vi "actuate_PairedPulseExp_v0.04.vi"(0 "Phase Cluster":T4, 1 "valve Time Cluster":T3, 2 "Didn't Lift?":bool, 3 "data in":T5={"daq_ao 1"="Dev1/ao0", "daq_ai 1"="Dev1/ai0", "experiment day folder"=path "D:/DATA/8-27-15 save func testing/test.lvm", "Multiclamp init error"=0, "Multiclamp Handle Out"=0, "sampling rate (Hz)"=10000, "trial name"=""}, 5 "PhaseLetter":string, 7 "controls array in":refnum<vi>[](array[refnum]), 9 "time to wait for solution change (min)":dbl=2.5 min=0.0 step=0.01, 11 "error in":errorcluster, 12 "common cluster":T7, 13 "individual controls in":T6) -> (4 "output cluster":T1, 6 "protocol waveform":waveform(dbl)[](graph), 8 "jumptestMonitor":waveform(dbl)[](graph) caption="protocol response", 10 "control array out":refnum<vi>[](array[refnum]), 14 "experiment VI ref":refnum<vi>, 15 "error out":errorcluster)   [LabVIEW 2019]
uses:
  pipette cleaning/pressure box/cleaning_soft/controls/actuator_type.ctl
  pipette cleaning/pressure box/cleaning_soft/controls/actuator_cluster.ctl
  machine_vision/coordinate model vis/transform_properties_actuators.ctl
  machine_vision/controls/transform_cluster_actuator.ctl
  controls/NH_method.ctl
  pipette cleaning/pressure box/cleaning_soft/controls/pressure_box_type.ctl
  pipette cleaning/pressure box/cleaning_soft/controls/pressure_box_control.ctl
  multipatch/controls/multipatch_common_controls_v4.ctl
  controls/memtest_def.ctl
  multipatch/controls/multipatch_individual_controls_v5.ctl
  Controls/Data.ctl
panel:
  in  "PairedPulseValuesCluster":T2
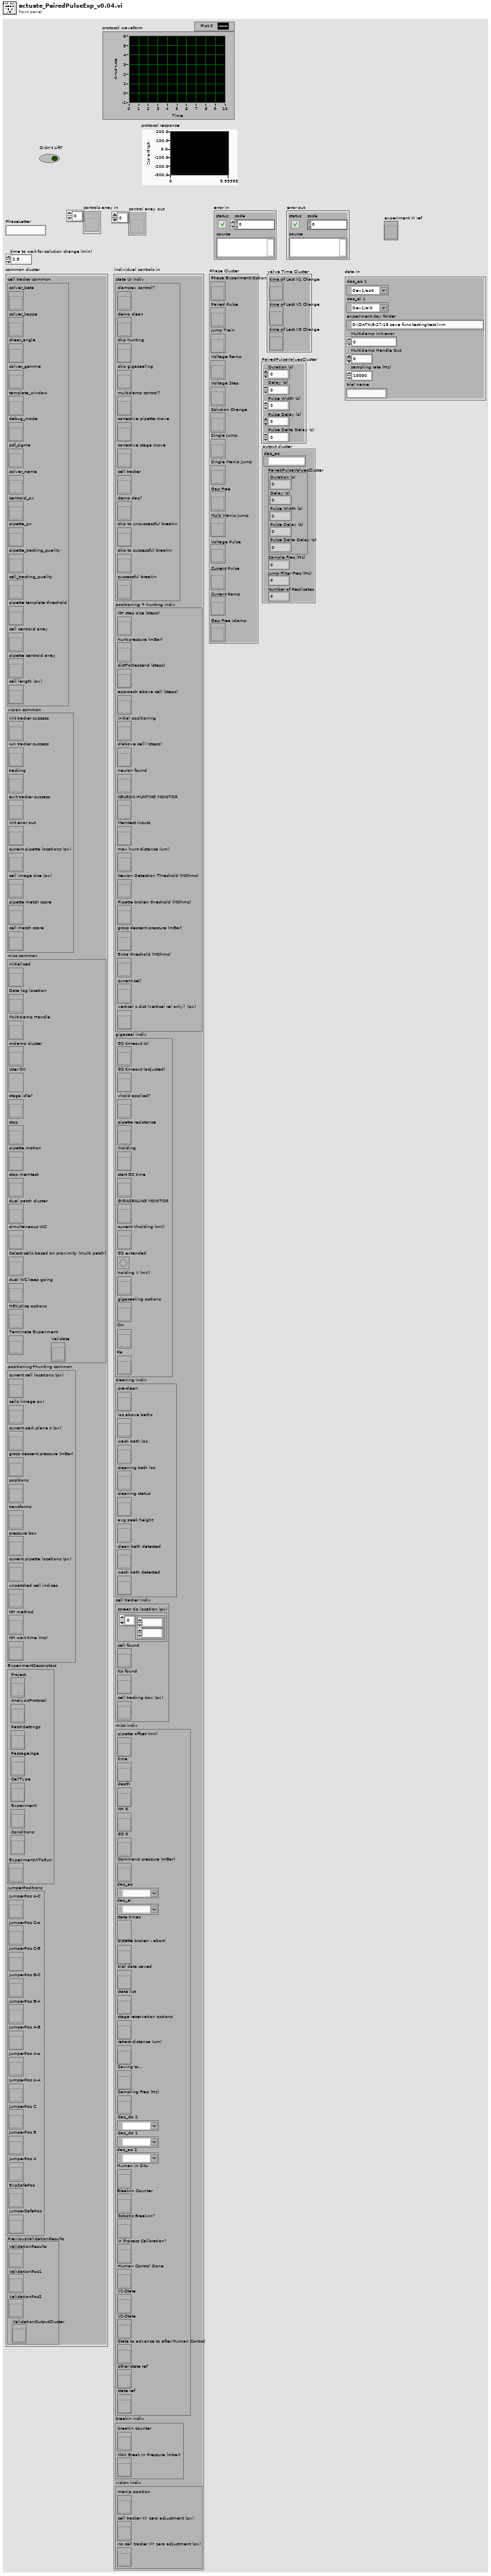
[diagram p1: front panel]
types:
  T1 = cluster{"daq_ao":tag, "PairedPulseValuesCluster":cluster{"Duration (s)":dbl, "Delay (s)":dbl, "Pulse Width (s)":dbl, "Pulse Delay (s)":dbl, "Pulse Delta Delay (s)":dbl}, "Sample Freq (Hz)":dbl, "Jump Filter Freq (Hz)":dbl, "Number of Replicates":i16}
  T2 = cluster{"Duration (s)":dbl, "Delay (s)":dbl, "Pulse Width (s)":dbl, "Pulse Delay (s)":dbl, "Pulse Delta Delay (s)":dbl}
  T3 = cluster{"time of Last V1 Change":refnum<vi>, "time of Last V2 Change":refnum<vi>, "time of Last V3 Change":refnum<vi>}
  T4 = cluster{"Phase Experiment Option":refnum<vi>, "Paired Pulse":refnum<vi>, "Jump Train":refnum<vi>, "Voltage Ramp":refnum<vi>, "Voltage Step":refnum<vi>, "Solution Change":refnum<vi>, "Single Jump":refnum<vi>, "Single Manip Jump":refnum<vi>, "Gap Free":refnum<vi>, "Multi Manip Jump":refnum<vi>, "Voltage Pulse":refnum<vi>, "Current Pulse":refnum<vi>, "Current Ramp":refnum<vi>, "Gap Free Iclamp":refnum<vi>}
  T5 = typedef "Data.ctl" = cluster{"daq_ao 1":tag, "daq_ai 1":tag, "experiment day folder":path, "Multiclamp init error":i32, "Multiclamp Handle Out":u32, "sampling rate (Hz)":i32, "trial name":string}
  T6 = typedef "multipatch_individual_controls_v5.ctl" = cluster{"state UI indiv":cluster{"clampex control?":refnum<vi>, "demo clean":refnum<vi>, "skip hunting":refnum<vi>, "skip gigasealing":refnum<vi>, "multiclamp control?":refnum<vi>, "corrective pipette move":refnum<vi>, "corrective stage move":refnum<vi>, "cell tracker":refnum<vi>, "demo daq?":refnum<vi>, "skip to unsuccessful breakin":refnum<vi>, "skip to successful breakin":refnum<vi>, "successful breakin":refnum<vi>}, "positioning + hunting indiv":cluster{"NH step size (steps)":refnum<vi>, "hunt pressure (mBar)":refnum<vi>, "distToDescend (steps)":refnum<vi>, "approach above cell (steps)":refnum<vi>, "initial positioning":refnum<vi>, "d(above cell) (steps)":refnum<vi>, "neuron found":refnum<vi>, "NEURON HUNTING MONITOR":refnum<vi>, "Memtest inputs":refnum<vi>, "max hunt distance (um)":refnum<vi>, "Neuron Detection Threshold (MOhms)":refnum<vi>, "Pipette broken threshold (MOhms)":refnum<vi>, "gross descent pressure (mBar)":refnum<vi>, "Extra threshold (MOhms)":refnum<vi>, "current cell":refnum<vi>, "vertical z dist (vertical rel only)  (px)":refnum<vi>}, "gigaseal indiv":cluster{"GS timeout (s)":refnum<vi>, "GS timeout (adjusted)":refnum<vi>, "vhold applied?":refnum<vi>, "pipette resistance":refnum<vi>, "Iholding":refnum<vi>, "start GS time":refnum<vi>, "GIGASEALING MONITOR":refnum<vi>, "current Vholding (mV)":refnum<vi>, "GS extended":refnum<vi>, "holding V (mV)":refnum<vi>, "gigasealing options":refnum<vi>, "Cm":refnum<vi>, "Ra ":refnum<vi>}, "cleaning indiv":cluster{"pre-clean":refnum<vi>, "loc above baths":refnum<vi>, "wash bath loc":refnum<vi>, "cleaning bath loc":refnum<vi>, "cleaning status":refnum<vi>, "avg peak height":refnum<vi>, "clean bath detected":refnum<vi>, "wash bath detected":refnum<vi>}, "cell tracker indiv":cluster{"screen tip location (px)":refnum<vi>, "cell found":refnum<vi>, "tip found":refnum<vi>, "cell tracking box (px)":refnum<vi>}, "misc indiv":cluster{"pipette offset (mV)":refnum<vi>, "time":refnum<vi>, "depth":refnum<vi>, "NH R":refnum<vi>, "GS R":refnum<vi>, "Command pressure (mBar)":refnum<vi>, "daq_ao":tag, "daq_ai":tag, "state times":refnum<vi>, "pipette broken - abort!":refnum<vi>, "trial data saved":refnum<vi>, "state list":refnum<vi>, "stage reservation options":refnum<vi>, "retract distance (um)":refnum<vi>, "Saving to...":refnum<vi>, "Sampling Freq (Hz)":refnum<vi>, "daq_do 2":tag, "daq_do 1":tag, "daq_ao 2":tag, "Human in Situ":refnum<vi>, "Break-In Counter":refnum<vi>, "Robotic Break-In?":refnum<vi>, "In Process Calibration?":refnum<vi>, "Human Control Done":refnum<vi>, "V1-State":refnum<vi>, "V2-State":refnum<vi>, "State to advance to after Human Control":refnum<vi>, "other state ref":refnum<vi>, "state ref":refnum<vi>}, "breakin indiv":cluster{"breakin counter":refnum<vi>, "MAX Break In Pressure (mbar)":refnum<vi>}, "vision indiv":cluster{"manip position":refnum<vi>, "cell tracker XY zero adjustment (px)":refnum<vi>, "no cell tracker XY zero adjustment (px)":refnum<vi>}}
  T7 = typedef "multipatch_common_controls_v4.ctl" = cluster{"cell tracker common":cluster{"solver_beta":refnum<vi>, "solver_kappa":refnum<vi>, "shear_angle":refnum<vi>, "solver_gamma":refnum<vi>, "template_window":refnum<vi>, "debug_mode":refnum<vi>, "psf_sigma":refnum<vi>, "solver_name":refnum<vi>, "centroid_px":refnum<vi>, "pipette_px":refnum<vi>, "pipette_tracking_quality":refnum<vi>, "cell_tracking_quality":refnum<vi>, "pipette template threshold":refnum<vi>, "cell centroid array":refnum<vi>, "pipette centroid array":refnum<vi>, "cell length (px)":refnum<vi>}, "vision common":cluster{"init tracker success":refnum<vi>, "run tracker success":refnum<vi>, "tracking":refnum<vi>, "exit tracker success":refnum<vi>, "init error out":refnum<vi>, "current pipette locations (px)":refnum<vi>, "cell image size (px)":refnum<vi>, "pipette match score":refnum<vi>, "cell match score":refnum<vi>}, "misc common":cluster{"initialized":refnum<vi>, "Data log location":refnum<vi>, "Multiclamp Handle":refnum<vi>, "mclamp cluster":refnum<vi>, "User OK":refnum<vi>, "stage idle?":refnum<vi>, "stop":refnum<vi>, "pipette motion":refnum<vi>, "stop memtest":refnum<vi>, "dual patch cluster":refnum<vi>, "simultaneous WC":refnum<vi>, "Select cells based on proximity (multi patch)":refnum<vi>, "dual WC keep going":refnum<vi>, "HEK/slice options":refnum<vi>, "Terminate Experiment":refnum<vi>, "Validate":refnum<vi>}, "positioning+hunting common":cluster{"current cell locations (px)":refnum<vi>, "cells (image px)":refnum<vi>, "current park plane z (px)":refnum<vi>, "gross descent pressure (mBar)":refnum<vi>, "positions":refnum<vi>, "transforms":refnum<vi>, "pressure box":refnum<vi>, "current pipette locations (px)":refnum<vi>, "unpatched cell indices":refnum<vi>, "NH method":refnum<vi>, "NH wait time (ms)":refnum<vi>}, "ExperimentDescriptors":cluster{"Project":refnum<vi>, "AnalysisProtocol":refnum<vi>, "PatchSettings":refnum<vi>, "Passage/Age":refnum<vi>, "CellType":refnum<vi>, "Experiment":refnum<vi>, "Conditions":refnum<vi>, "ExperimentVIToRun":refnum<vi>}, "JumperPositions":cluster{"JumperPos o-C":refnum<vi>, "JumperPos C-o":refnum<vi>, "JumperPos C-B":refnum<vi>, "JumperPos B-C":refnum<vi>, "JumperPos B-A":refnum<vi>, "JumperPos A-B":refnum<vi>, "JumperPos A-o":refnum<vi>, "JumperPos o-A":refnum<vi>, "JumperPos C":refnum<vi>, "JumperPos B":refnum<vi>, "JumperPos A":refnum<vi>, "ExpSafePos":refnum<vi>, "jumperSafePos":refnum<vi>}, "PreviousValidationResults":cluster{"ValidationResults":refnum<vi>, "ValidationPos1":refnum<vi>, "ValidationPos2":refnum<vi>, "ValidationOutputCluster":refnum<vi>}}
  T8 = cluster{"Which Position to use for Experiment":enum16{"Jumper Safe Position", "Experiment Safe Position", "Jumper Position A", "Jumper Position B", "Jumper Position C", "Jumper Position o-A", "Jumper Position A-o", "Jumper Position A-B", "Jumper Position B-A", "Jumper Position B-C", "Jumper Position C-B", "Jumper Position C-o", "Jumper Position o-C", "Don't Move"}, "Start Position (N)":string, "Jump Position (m)":string, "Duration (s)":dbl, "Delay (s)":dbl, "Pulse Width (s)":dbl, "Replicates":dbl, "Pulse Delay (s)":dbl, "Pulse Delta Delay (s)":dbl, "Vholding (mV)":dbl, "Valve 1 Position":i16, "Valve 2 Position":i16, "valve 1 used now?":bool, "valve 2 used now?":bool, "valve 3 used now? ":bool, "Valve 3 Position":i16, "protocol Preview":waveform(dbl)[]}
  T9 = enum16{"Jumper Safe Position", "Experiment Safe Position", "Jumper Position A", "Jumper Position B", "Jumper Position C", "Jumper Position o-A", "Jumper Position A-o", "Jumper Position A-B", "Jumper Position B-A", "Jumper Position B-C", "Jumper Position C-B", "Jumper Position C-o", "Jumper Position o-C", "Don't Move"}
  T10 = enum16{"manipulator 1", "manipulator 2", "manipulator 3", "manipulator 4"}
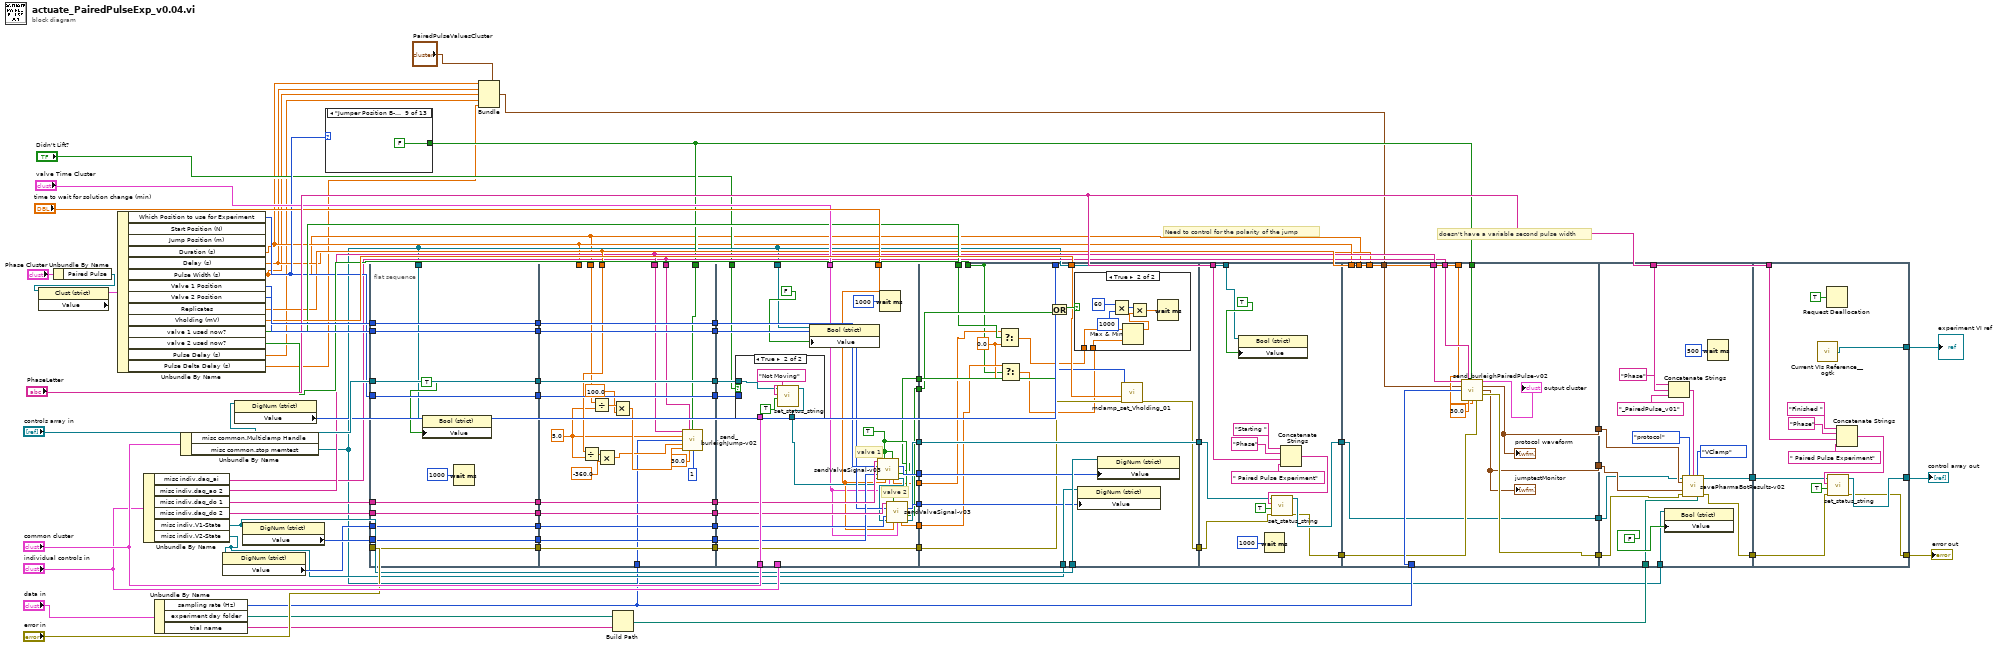
[diagram p0: block diagram]
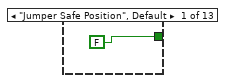
[diagram p2: hidden frame]
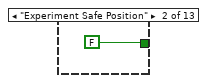
[diagram p3: hidden frame]
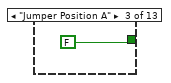
[diagram p4: hidden frame]
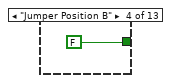
[diagram p5: hidden frame]
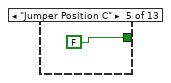
[diagram p6: hidden frame]
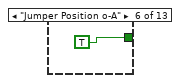
[diagram p7: hidden frame]
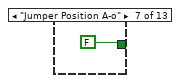
[diagram p8: hidden frame]
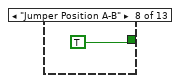
[diagram p9: hidden frame]
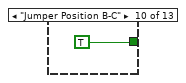
[diagram p10: hidden frame]
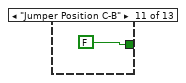
[diagram p11: hidden frame]
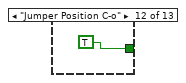
[diagram p12: hidden frame]
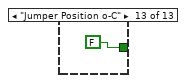
[diagram p13: hidden frame]
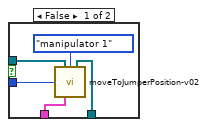
[diagram p14: hidden frame]
diagram:
  # "doesn't have a variable second pulse width"
  # "Need to control for the polarity of the jump"
  n1 = Unbundle By Name("Phase Cluster") -> ("Paired Pulse"=w59:refnum<vi>)
  n2 = property class="Clust (strict)"(reference=w59) -> ("Value"=w58:T8)  [unwired: 1 in, 2 out]
  n3 = Unbundle By Name(w58) -> ("Which Position to use for Experiment"=w34:T9, "Duration (s)"=w8:dbl, "Delay (s)"=w7:dbl, "Pulse Width (s)"=w6:dbl, "Valve 1 Position"=w57:i16, "Valve 2 Position"=w56:i16, "Replicates"=w24:dbl, "Vholding (mV)"=w43:dbl, "valve 1 used now?"=w36:bool, "valve 2 used now?"=w35:bool, "Pulse Delay (s)"=w5:dbl, "Pulse Delta Delay (s)"=w4:dbl)  [unwired: 2 out]
  n4 = Unbundle By Name("individual controls in") -> ("misc indiv.daq_ai"=w21:tag, "misc indiv.daq_ao 2"=w22:tag, "misc indiv.daq_do 1"=w79:tag, "misc indiv.daq_do 2"=w78:tag, "misc indiv.V1-State"=w70:refnum<vi>, "misc indiv.V2-State"=w69:refnum<vi>)
  n5 = Unbundle By Name("data in") -> ("sampling rate (Hz)"=w23:i32, "experiment day folder"=w63:path, "trial name"=w62:string)
  n6 = Unbundle By Name("common cluster") -> ("misc common.Multiclamp Handle"=w42:refnum<vi>, "misc common.stop memtest"=w10:refnum<vi>)
  n7 = property class="DigNum (strict)"(reference=w69) -> ("Value"=w71:u16)  [unwired: 1 in, 2 out]
  n8 = property class="DigNum (strict)"(reference=w42) -> ("Value"=w41:u32)  [unwired: 1 in, 2 out]
  n9 = property class="DigNum (strict)"(reference=w70) -> ("Value"=w72:u16)  [unwired: 1 in, 2 out]
  n10 = case shown="\"Jumper Position B-A\"" w34 {
    tunnel: [FALSE FALSE FALSE FALSE FALSE TRUE FALSE TRUE FALSE TRUE FALSE TRUE FALSE] -> w20
    frame "Jumper Safe Position", Default {
    }
    frame "Experiment Safe Position" {
    }
    frame "Jumper Position A" {
    }
    frame "Jumper Position B" {
    }
    frame "Jumper Position C" {
    }
    frame "Jumper Position o-A" {
    }
    frame "Jumper Position A-o" {
    }
    frame "Jumper Position A-B" {
    }
    frame "Jumper Position B-A" {
    }
    frame "Jumper Position B-C" {
    }
    frame "Jumper Position C-B" {
    }
    frame "Jumper Position C-o" {
    }
    frame "Jumper Position o-C" {
    }
  }
  n11 = flat-sequence {
    tunnel: "controls array in" -> [w98]
    tunnel: w56 -> [w99]
    tunnel: w57 -> [w100]
    tunnel: w71 -> [w101]
    tunnel: w72 -> [w102]
    tunnel: "error in" -> [w103]
    tunnel: w78 -> [w104]
    tunnel: w79 -> [w105]
    tunnel: w34 -> [w106]
    tunnel: [w106] -> w19
    tunnel: [w105] -> w18
    tunnel: [w104] -> w17
    tunnel: [w103] -> w16
    tunnel: [w102] -> w15
    tunnel: [w101] -> w14
    tunnel: [w100] -> w13
    tunnel: [w99] -> w12
    tunnel: [w98] -> w11
    tunnel: w10 -> [w96]
    tunnel: [w130] -> w33
    tunnel: [w129] -> w32
    tunnel: [w128] -> w31
    tunnel: [w127] -> w30
    tunnel: [w126] -> w29
    tunnel: [w125] -> w28
    tunnel: [w124] -> w27
    tunnel: [w123] -> w26
    tunnel: [w122] -> w25
    tunnel: w8 -> [_]
    tunnel: w24 -> [w115]
    tunnel: w6 -> [w114]
    tunnel: w23 -> [w113]
    tunnel: w22 -> [w112]
    tunnel: w21 -> [w111]
    tunnel: w20 -> [w109]
    tunnel: w19 -> [w130]
    tunnel: w18 -> [w129]
    tunnel: w17 -> [w128]
    tunnel: w16 -> [w127]
    tunnel: w15 -> [w126]
    tunnel: w14 -> [w125]
    tunnel: w13 -> [w124]
    tunnel: w12 -> [w123]
    tunnel: w11 -> [w122]
    tunnel: "common cluster" -> [w155]
    tunnel: "individual controls in" -> [_]
    tunnel: [w152] -> w74
    tunnel: [w149] -> w68
    tunnel: [w148] -> w67
    tunnel: [w142] -> w50
    tunnel: [w140] -> w45
    tunnel: [w139] -> w44
    tunnel: "time to wait for solution change (min)" -> [w138]
    tunnel: "valve Time Cluster" -> [w137]
    tunnel: [w136] -> w38
    tunnel: [w135] -> w37
    tunnel: w33 -> [w156]
    tunnel: w32 -> [w154]
    tunnel: w31 -> [w153]
    tunnel: w30 -> [w152]
    tunnel: w29 -> [w151]
    tunnel: w28 -> [w150]
    tunnel: w27 -> [w147]
    tunnel: w26 -> [w146]
    tunnel: w25 -> [w145]
    tunnel: w10 -> [w133]
    tunnel: "Didn't Lift?" -> [w131]
    tunnel: [w173] -> w75
    tunnel: w74 -> [w175]
    tunnel: w70 -> [w184]
    tunnel: w69 -> [w183]
    tunnel: w68 -> [w182]
    tunnel: w67 -> [w181]
    tunnel: [w180] -> w51
    tunnel: w50 -> [w180]
    tunnel: w45 -> [w178]
    tunnel: w44 -> [w177]
    tunnel: w43 -> [w176]
    tunnel: w41 -> [w174]
    tunnel: w38 -> [w170]
    tunnel: w37 -> [w169]
    tunnel: w36 -> [w171]
    tunnel: [w166] -> _
    tunnel: w35 -> [w166]
    tunnel: w10 -> [w192]
    tunnel: [w194] -> w76
    tunnel: w75 -> [w195]
    tunnel: [w196] -> w52
    tunnel: w51 -> [w197]
    tunnel: "PhaseLetter" -> [w198]
    tunnel: w21 -> [w216]
    tunnel: w22 -> [w215]
    tunnel: w76 -> [w210]
    tunnel: [w213] -> w66
    tunnel: [w207] -> w65
    tunnel: w24 -> [w211]
    tunnel: w8 -> [_]
    tunnel: w23 -> [w212]
    tunnel: w6 -> [_]
    tunnel: w7 -> [_]
    tunnel: [w209] -> w55
    tunnel: [w208] -> w53
    tunnel: w52 -> [w208]
    tunnel: w20 -> [w206]
    tunnel: w3 -> [w205]
    tunnel: w10 -> [w232]
    tunnel: w66 -> [w231]
    tunnel: w65 -> [w230]
    tunnel: w61 -> [w227]
    tunnel: "PhaseLetter" -> [w225]
    tunnel: w55 -> [w222]
    tunnel: w53 -> [w221]
    tunnel: [w219] -> w48
    tunnel: [w220] -> w47
    tunnel: [w239] -> w49
    tunnel: [w238] -> w73
    tunnel: w48 -> [w237]
    tunnel: w47 -> [w240]
    tunnel: "PhaseLetter" -> [w236]
    tunnel: [w235] -> w1
    frame #0 {
      n12 = property class="Bool (strict)"(reference=w96, "Value"=TRUE ("stop memtest")) -> ()  [unwired: 1 in, 2 out]
      n13 = Wait (ms)(milliseconds to wait=u32 1000) -> ()  [unwired: 1 out]
    }
    frame #1 {
      w107 = 5.0 ("y")
      n14 = Divide(x=w115, y=w107) -> (x/y=w117:dbl)
      n15 = Divide(x=w114, y=w107) -> (x/y=w120:dbl)
      n16 = Multiply(x=w117, y=-360.0) -> (x*y=w116:dbl)
      n17 = Multiply(x=w120, y=100.0) -> (x*y=w118:dbl)
      n18 = call "send_burleighJump-v02.vi"("daq_ao 2"=w112, "daq_ai"=w111, "Jump Polarity"=w109, "Duration (s)"=w107, "Sample Freq (Hz)"=w113, "Phase"=w116, "Duty Cycle"=w118, "Jump Filter Freq (Hz)"=30.0, "Number of Replicates"=i16 1) -> ()  [unwired: 3 in, 4 out]
    }
    frame #2 {
      w141 = TRUE ("Set Status")
      # "valve 2"
      # "valve 1"
      n19 = case shown="True" w131 {
        tunnel: w156 -> [w161 _]
        tunnel: w155 -> [w160 _]
        tunnel: w145 -> [w158 w162]
        tunnel: [w157 w163] -> w144
        frame False {
          n20 = call "moveToJumperPosition-v02.vi"("which manipulator"=T10."manipulator 1", "controls array in"=w158, "Which Jumper Position to move to?"=w161, "common cluster"=w160) -> ("control array out"=w157:refnum<vi>[])  [unwired: 10 in, 1 out]
        }
        frame True {
          n21 = call "set_status_string.vi"("new line?"=TRUE, "status string in"="Not Moving", "controls array"=w162) -> ("controls array out"=w163:refnum<vi>[])  [unwired: 7 in, 1 out]
        }
      }
      n22 = property class="Bool (strict)"(reference=w133, "Value"=FALSE ("stop memtest")) -> ()  [unwired: 1 in, 2 out]
      n23 = call "sendValveSignal-v03.vi"("daq_do"=w154, "Set Status"=w141, "Valve1?"=w141, "ChangeToValve"=w147, "CurrentValve"=w151, "controls array in"=w144, "time to wait for solution change (min)"=w138, "valve Time Cluster"=w137) -> ("ValveSetTo"=w148:u16, "valve changed?"=w140:bool, "additional time to wait (min)"=w136:dbl, "control array out"=w143:refnum<vi>[])  [unwired: 4 in]
      n24 = Wait (ms)(milliseconds to wait=u32 1000) -> ()  [unwired: 1 out]
      n25 = call "sendValveSignal-v03.vi"("daq_do"=w153, "Set Status"=w141, "ChangeToValve"=w146, "CurrentValve"=w150, "controls array in"=w143, "time to wait for solution change (min)"=w138, "valve Time Cluster"=w137) -> ("ValveSetTo"=w149:u16, "valve changed?"=w139:bool, "additional time to wait (min)"=w135:dbl, "control array out"=w142:refnum<vi>[])  [unwired: 5 in]
    }
    frame #3 {
      w167 = 0.0 ("f")
      n26 = Select(t=w170, s=w171, f=w167) -> (s? t:f=w172:dbl)
      n27 = Select(t=w169, s=w166, f=w167) -> (s? t:f=w168:dbl)
      n28 = Or(x=w178, y=w177) -> (x .or. y?=w179:bool)
      n29 = case shown="True" w179 {
        tunnel: w172 -> [_ w187]
        tunnel: w168 -> [_ w186]
        frame False {
        }
        frame True {
          n30 = Multiply(x=u32 60 ("milliseconds to wait"), y=u32 1000) -> (x*y=w189:u32)
          n31 = Max & Min(x=w187, y=w186) -> (max(x,y)=w185:dbl)  [unwired: 1 out]
          n32 = Multiply(x=w189, y=w185) -> (x*y=w188:dbl)
          n33 = Wait (ms)(milliseconds to wait=w188) -> ()  [unwired: 1 out]
        }
      }
      n34 = property class="DigNum (strict)"(reference=w183, "Value"=w182) -> ()  [unwired: 1 in, 2 out]
      n35 = property class="DigNum (strict)"(reference=w184, "Value"=w181) -> ()  [unwired: 1 in, 2 out]
      n36 = call "mclamp_set_Vholding_01.vi"("error in (no error)"=w175, "set holding (mV)"=w176, "Multiclamp Handle Out"=w174) -> ("error out"=w173:errorcluster)  [unwired: 7 in, 1 out]
    }
    frame #4 {
      n37 = property class="Bool (strict)"(reference=w192, "Value"=TRUE ("stop memtest")) -> ()  [unwired: 1 in, 2 out]
      n38 = Wait (ms)(milliseconds to wait=u32 1000) -> ()  [unwired: 1 out]
      n39 = Concatenate Strings("Starting " ("string"), "Phase" ("string"), w198, " Paired Pulse Experiment" ("string")) -> (w200:string)
      n40 = call "set_status_string.vi"("error in"=w195, "new line?"=TRUE, "status string in"=w200, "controls array"=w197) -> ("error out"=w194:errorcluster, "controls array out"=w196:refnum<vi>[])  [unwired: 6 in]
    }
    frame #5 {
      n41 = call "send_burleighPairedPulse-v02.vi"("daq_ao"=w215, "daq_ai"=w216, "Jump Polarity"=w206, "PairedPulseValuesCluster"=w205, "Sample Freq (Hz)"=w212, "Jump Filter Freq (Hz)"=30.0, "Number of Replicates"=w211, "error in"=w210) -> ("output cluster"=→"output cluster":T1, "output waveform"=w213:waveform(dbl)[], "protocol response"=w207:waveform(dbl)[], "error out"=w209:errorcluster)  [unwired: 4 in]
      "jumptestMonitor" <- w207
      "protocol waveform" <- w213
    }
    frame #6 {
      n42 = property class="Bool (strict)"(reference=w232, "Value"=FALSE ("stop memtest")) -> ()  [unwired: 1 in, 2 out]
      n43 = Concatenate Strings("Phase" ("string"), w225, "_PairedPulse_v01" ("string")) -> (w226:string)
      n44 = call "savePharmaBotResults-v02.vi"("controls array"=w221, "protocol or memtest"=enum16{"protocol", "memtest", "validation"}."protocol", "ExpPhase"=w226, "which clamp"=enum16{"VClamp", "IClamp"}."VClamp", "protocol waveform"=w231, "protocol response"=w230, "error in"=w222, "Save to (folder dir)"=w227) -> ("controls array out"=w220:refnum<vi>[], "error out"=w219:errorcluster)  [unwired: 6 in]
      n45 = Wait (ms)(milliseconds to wait=u32 500) -> ()  [unwired: 1 out]
    }
    frame #7 {
      n46 = call "Current VIs Reference__ogtk.vi"() -> ("Current VI's reference"=w235:refnum<vi>)  [unwired: 5 in]
      n47 = Request Deallocation(TRUE ("flag")) -> ()
      n48 = Concatenate Strings("Finished " ("string"), "Phase" ("string"), w236, " Paired Pulse Experiment" ("string")) -> (w242:string)
      n49 = call "set_status_string.vi"("error in"=w237, "new line?"=TRUE, "status string in"=w242, "controls array"=w240) -> ("error out"=w238:errorcluster, "controls array out"=w239:refnum<vi>[])  [unwired: 6 in]
    }
  }
  n50 = Bundle(cluster="PairedPulseValuesCluster", "Duration (s)"=w8, "Delay (s)"=w7, "Pulse Width (s)"=w6, "Pulse Delay (s)"=w5, "Pulse Delta Delay (s)"=w4) -> (w3:T2)
  n51 = Build Path(base path=w63, name or relative path=w62) -> (appended path=w61:path)
  "error out" <- w73
  "control array out" <- w49
  "experiment VI ref" <- w1
